vi "Configure Histogram.vi"(0 "VISA resource name":refnum<visa-resource-name>, 1 "Enable Histogram (Yes)":bool=TRUE, 2 "Reset (ON)":bool=TRUE, 5 "Channels (0:Channel1)":u16(ring) items=["Channel 1", "Channel 2", "Channel 3", "Channel 4", "Math 1", "Math 2", "Math 3", "Math 4", "Reference 1", "Reference 2", "Reference 3", "Reference 4"], 7 "Histogram Type (0:Horizontal)":u16(ring) items=["Horizontal", "Vertical"], 9 "Histogram Scaling (0:Linear)":u16(ring) items=["Linear", "Log"], 11 "error in (no error)":errorcluster, 12 "Adjust Histogram Box":T1={"Left Limit (-0.001s)"=-0.001, "Top Limit (1.25V)"=1.25, "Right Limit (0.001s)"=0.001, "Bottom Limit (-1.25v)"=-1.25}) -> (4 "VISA resource name out":refnum<visa-resource-name>, 15 "error out":errorcluster)   [LabVIEW 2011, in "Tektronix 7000 Series.lvlib"]
doc: "Configures the Histogram properties of an oscilloscope. You can configure the Histogram Type, Scaling Type and so on."
uses:
  Tektronix 7000 Series.lvlib
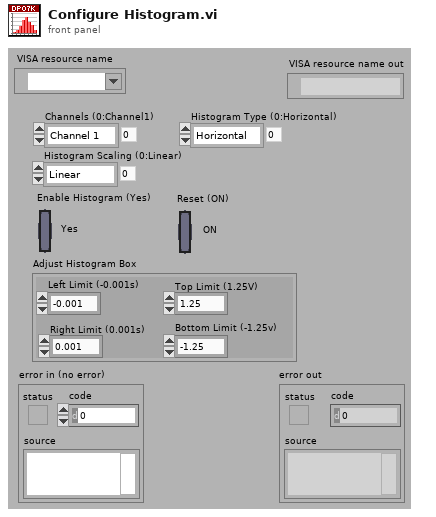
[diagram p1: front panel]
types:
  T1 = cluster{"Left Limit (-0.001s)":dbl, "Top Limit (1.25V)":dbl, "Right Limit (0.001s)":dbl, "Bottom Limit (-1.25v)":dbl}
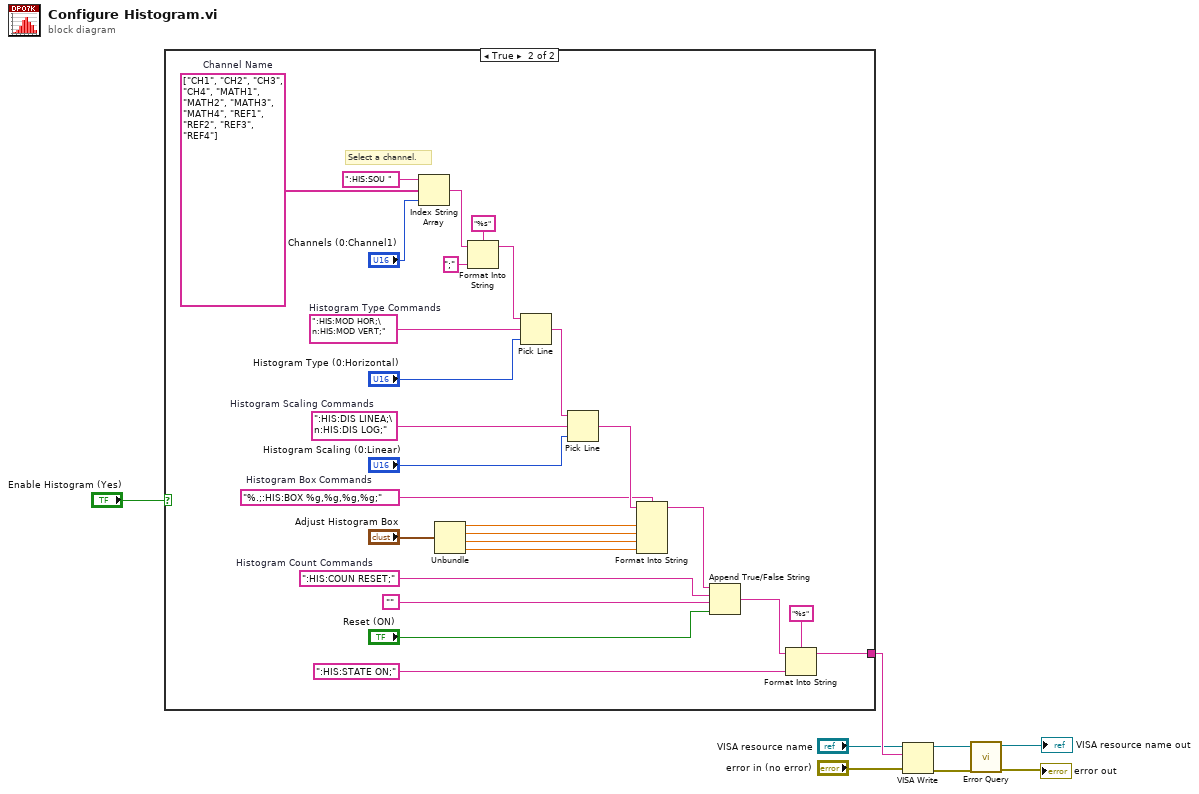
[diagram p0: block diagram]
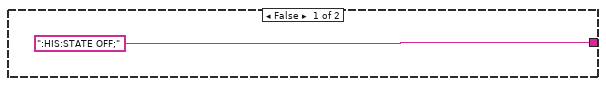
[diagram p2: hidden frame]
diagram:
  n1 = case shown="True" "Enable Histogram (Yes)" {
    tunnel: [":HIS:STATE OFF;" w14] -> w7
    frame False {
    }
    frame True {
      w19 = ":HIS:COUN RESET;"  # Histogram Count Commands
      w22 = string[] ["CH1", "CH2", "CH3", "CH4", "MATH1", "MATH2", "MATH3", "MATH4", "REF1", "REF2", "REF3", "REF4"]  # Channel Name
      w25 = "%.;:HIS:BOX %g,%g,%g,%g;"  # Histogram Box Commands
      w34 = ":HIS:DIS LINEA;\n:HIS:DIS LOG;"  # Histogram Scaling Commands
      w36 = ":HIS:MOD HOR;\n:HIS:MOD VERT;"  # Histogram Type Commands
      # "Select a channel."
      n2 = Index String Array(1:"Channels (0:Channel1)", 2:w22, 3:":HIS:SOU " ("format string")) -> (0:w11:string)
      n3 = Unbundle("Adjust Histogram Box") -> ("Left Limit (-0.001s)"=w29:dbl, "Top Limit (1.25V)"=w28:dbl, "Right Limit (0.001s)"=w27:dbl, "Bottom Limit (-1.25v)"=w26:dbl)
      n4 = Format Into String(format string="%s", initial string=w11, ";" ("input 1")) -> (resulting string=w10:string)  [unwired: 1 in, 1 out]
      n5 = Pick Line(string ("")=w10, multi-line string=w36, line index="Histogram Type (0:Horizontal)") -> (output string=w33:string)
      n6 = Pick Line(string ("")=w33, multi-line string=w34, line index="Histogram Scaling (0:Linear)") -> (output string=w30:string)
      n7 = Format Into String(format string=w25, initial string=w30, w29, w28, w27, w26) -> (resulting string=w20:string)  [unwired: 1 in, 1 out]
      n8 = Append True/False String(1:"Reset (ON)", 2:"" ("Empty String Constant"), 3:w19, 4:w20) -> (0:w15:string)
      n9 = Format Into String(format string="%s", initial string=w15, ":HIS:STATE ON;") -> (resulting string=w14:string)  [unwired: 1 in, 1 out]
    }
  }
  n10 = VISA Write(VISA resource name="VISA resource name", write buffer=w7, error in (no error)="error in (no error)") -> (VISA resource name out=w4:refnum<visa-resource-name>, error out=w3:errorcluster)  [unwired: 1 out]
  n11 = call "Error Query.vi"("error in (no error)"=w3, "VISA resource name"=w4) -> ("error out"=→"error out":errorcluster, "VISA resource name out"=→"VISA resource name out":refnum<visa-resource-name>)  [unwired: 6 in, 2 out]
